vi "Get Threads.vi"(7 "Base Threads":string[](array[string]), 8 "error in (no error)":errorcluster, 11 "App Reference":refnum<vi>) -> (0 "error out":errorcluster, 3 "Threads":string[](array[string]))   [LabVIEW 2017]
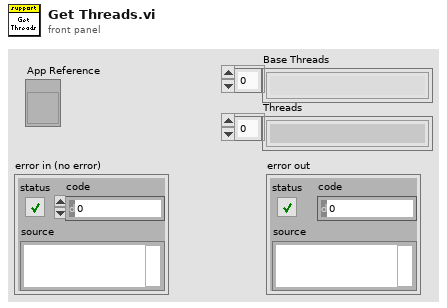
[diagram p1: front panel]
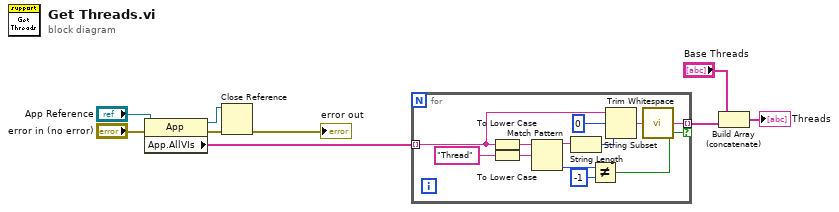
[diagram p0: block diagram]
diagram:
  n1 = property class="App"(reference="App Reference", error in="error in (no error)") -> (reference out=w3:refnum<vi>, error out=w6:errorcluster, "App.AllVIs"=w9:string[])
  n2 = Close Reference(reference=w3, error in (no error)=w6) -> (error out=→"error out":errorcluster)
  n3 = for {
    tunnel: w9 -> [w16] mode=indexing
    tunnel: [w10] -> w8 mode=indexing if=w11
    n4 = To Lower Case(string=w16) -> (all lower case string=w18:string)
    n5 = To Lower Case(string="Thread" ("regular expression")) -> (all lower case string=w17:string)
    n6 = Match Pattern(string=w18, regular expression=w17) -> (before substring=w15:string, offset past match=w20:i32)  [unwired: 1 in, 2 out]
    n7 = String Length(string=w15) -> (length=w14:i32)
    n8 = Not Equal?(x=w20, y=-1) -> (x != y?=w11:bool)
    n9 = String Subset(string=w16, offset (0)=0, length (rest)=w14) -> (substring=w12:string)
    n10 = call <vilib>:"Trim Whitespace.vi"("string"=w12) -> ("trimmed string"=w10:string)  [unwired: 1 in]
  }
  n11 = Build Array (concatenate)("Base Threads", w8) -> (→"Threads":string[])
